vi "Exersize 3-6.vi"() -> ()   [LabVIEW 2014]
panel:
  in  "Enum":T1(ring)
  in  "deg from":dbl
  out "deg to":dbl
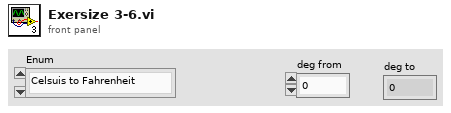
[diagram p1: front panel]
types:
  T1 = enum16{"Celsuis to Fahrenheit", "Fahrenheit to Celsius", "Celsuis to Kelvin", "Fahrenheit to Kelvin "}
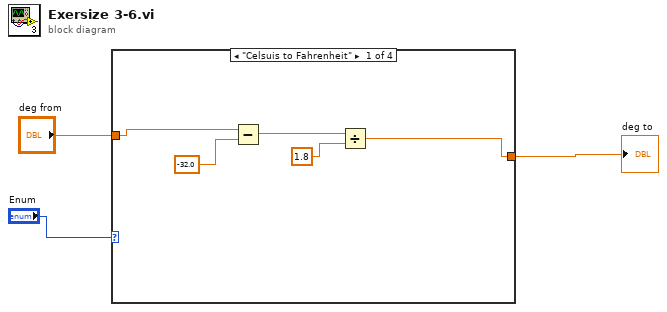
[diagram p0: block diagram]
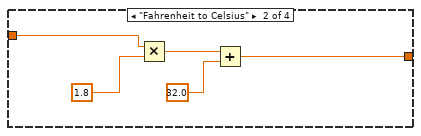
[diagram p2: hidden frame]
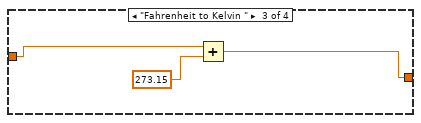
[diagram p3: hidden frame]
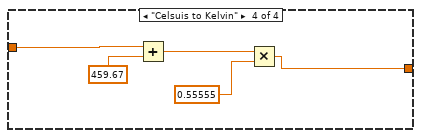
[diagram p4: hidden frame]
diagram:
  n1 = case shown="\"Celsuis to Fahrenheit\"" "Enum" {
    tunnel: "deg from" -> [w7 w10 w15 w21]
    tunnel: [w4 w9 w14 w17] -> w1
    frame "Celsuis to Fahrenheit" {
      n2 = Subtract(x=w7, y=-32.0) -> (x-y=w6:dbl)
      n3 = Divide(x=w6, y=1.8 ("x")) -> (x/y=w4:dbl)
    }
    frame "Fahrenheit to Celsius" {
      n4 = Multiply(x=w10, y=1.8) -> (x*y=w12:dbl)
      n5 = Add(x=w12, y=32.0) -> (x+y=w9:dbl)
    }
    frame "Fahrenheit to Kelvin " {
      n6 = Add(x=w15, y=273.15) -> (x+y=w14:dbl)
    }
    frame "Celsuis to Kelvin" {
      n7 = Add(x=w21, y=459.67) -> (x+y=w19:dbl)
      n8 = Multiply(x=w19, y=0.55555) -> (x*y=w17:dbl)
    }
  }
  "deg to" <- w1
